vi "Global VI.vi"() -> ()   [LabVIEW 2013]
uses:
  <vilib>/ActorFramework/Message Enqueuer/Message Enqueuer.lvclass
panel:
  in  "Message Array":refnum<class "Message Enqueuer.lvclass">[](array[class])
  out "test":dbl
  out "Card Cluster":T1
  in  "# Of Cards":i32
  in  "Data":dbl[](array[numeric])
  in  "VISA WT1600":refnum<visa-resource-name>
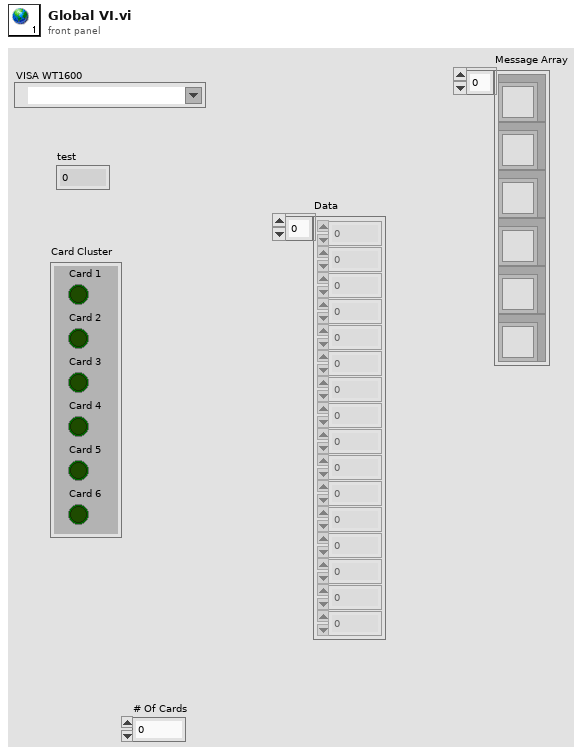
[diagram p1: front panel]
types:
  T1 = cluster{"Card 1":bool, "Card 2":bool, "Card 3":bool, "Card 4":bool, "Card 5":bool, "Card 6":bool}
diagram:
